vi "_ReadSpectralDataFile.vi"(0 "file path (dialog if empty)":path=path "C:/Users/Min/Projects/SVN/Sniffer900/Server/PeakDetection/Q1 PPG Pos IonSniffer-140926.txt") -> (1 "SpectralData":dbl[][](array[numeric]), 2 "Y":dbl[](array[numeric]), 3 "X":dbl[](array[numeric]))   [LabVIEW 2012]
uses:
  <vilib>/Utility/file.llb/Read From Spreadsheet File (DBL).vi
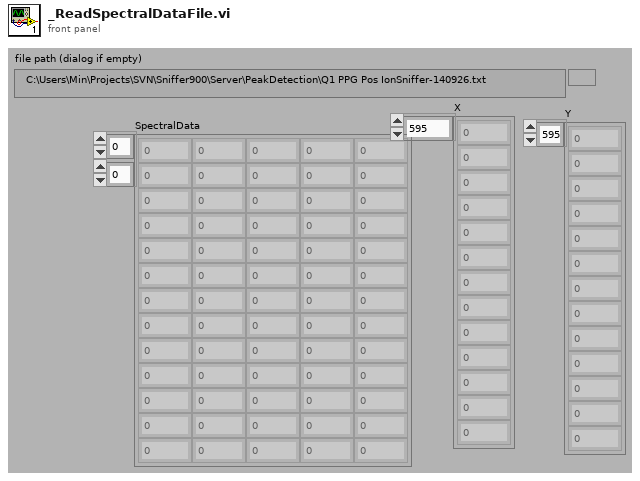
[diagram p1: front panel]
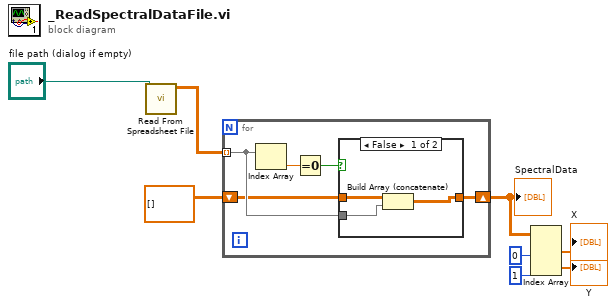
[diagram p0: block diagram]
diagram:
  n1 = call-poly <vilib>:"Read From Spreadsheet File.vi"("file path (dialog if empty)"="file path (dialog if empty)") -> ("all rows"=w7:dbl[][])  [unwired: 6 in, 4 out]
  n2 = for {
    tunnel: w7 -> [w11] mode=indexing
    shift-right: [w9] -> w5
    shift-left: dbl[][] [] ("all rows") -> [w10]
    n3 = Index Array(array=w11) -> (element=w13:dbl)  [unwired: 1 in]
    n4 = Equal To 0?(x=w13) -> (x = 0?=w12:bool)
    n5 = case shown="False" w12 {
      tunnel: w11 -> [w15 _]
      tunnel: w10 -> [w16 w17]
      tunnel: [w14 w17] -> w9
      frame False {
        n6 = Build Array (concatenate)(w16, w15) -> (w14:dbl[][])
      }
      frame True {
      }
    }
  }
  "SpectralData" <- w5
  n7 = Index Array(array=w5, index (col) #1=0 ("disabled index (col)"), index (col) #2=1 ("index (col)")) -> (element #1=→"X":dbl[], element #2=→"Y":dbl[])  [unwired: 2 in]
